vi "Update Stack Q.vi"(9 "Destination":dbl, 10 "Mode":enum16{"Add", "Replace"}(ring), 11 "Motor States":T1) -> ()   [LabVIEW 2016, in "Hardware.lvlib" / "Motions.lvlib" / "Motions.lvclass"]
uses:
  <userlib>/Common Components/Hardware/Abstract System/Motions/Motions/Motions.lvclass
  <userlib>/Common Components/Hardware/Abstract System/Motions/Motions/Motor States.ctl
  <userlib>/Common Components/TriggerAction Q/TriggerAction Q/TriggerAction Q.lvclass
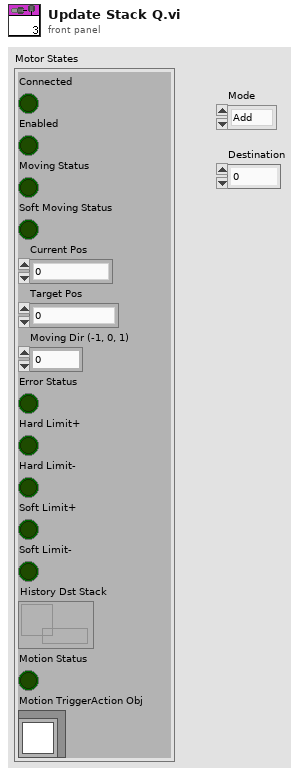
[diagram p1: front panel]
types:
  T1 = typedef "Hardware.lvlib/Motions.lvlib/Motions.lvclass/Motor States.ctl" = cluster{"Connected":bool, "Enabled":bool, "Moving Status":bool, "Soft Moving Status":bool, "Current Pos":dbl, "Target Pos":dbl, "Moving Dir (-1, 0, 1)":i32, "Error Status":bool, "Hard Limit+":bool, "Hard Limit-":bool, "Soft Limit+":bool, "Soft Limit-":bool, "History Dst Stack":refnum<queue>, "Motion Status":bool, "Motion TriggerAction Obj":refnum<class "TriggerAction Q.lvclass">}
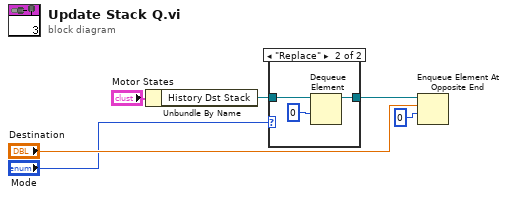
[diagram p0: block diagram]
diagram:
  n1 = Unbundle By Name("Motor States") -> ("History Dst Stack"=w3:refnum<queue>)
  n2 = case shown="\"Replace\"" "Mode" {
    tunnel: w3 -> [w7 w10]
    tunnel: [w7 w8] -> w5
    frame "Add", Default {
    }
    frame "Replace" {
      n3 = Dequeue Element(queue=w10, timeout in ms (-1)=0) -> (queue out=w8:refnum<queue>)  [unwired: 1 in, 3 out]
    }
  }
  n4 = Enqueue Element At Opposite End(queue=w5, element="Destination", timeout in ms (-1)=0) -> ()  [unwired: 1 in, 3 out]
